vi "plate tap.vi"() -> ()   [LabVIEW 2014]
uses:
  <vilib>/userdefined/High Color/IMAQdx.ctl
  <vilib>/Utility/file.llb/Write To Spreadsheet File (DBL).vi
  <vilib>/Utility/file.llb/Write To Spreadsheet File (string).vi
  <vilib>/vision/driver/NI_Vision_Acquisition_Software.lvlib
panel:
  in  "Tags":string
  in  "Hold Time (frames)":i32
  in  "ISI  (frames)":i32
  in  "Array":dbl[](array[numeric])
  in  "Trials Per Voltage":i32
  in  "Start Recording":bool
  in  "Min Voltage":dbl
  out "Frames":i32
  out "Error":string
  out "Save Directory":path
  out "Buffer Number Out":u32
  out "Image":T1(plugin-control)
  in  "stop":bool
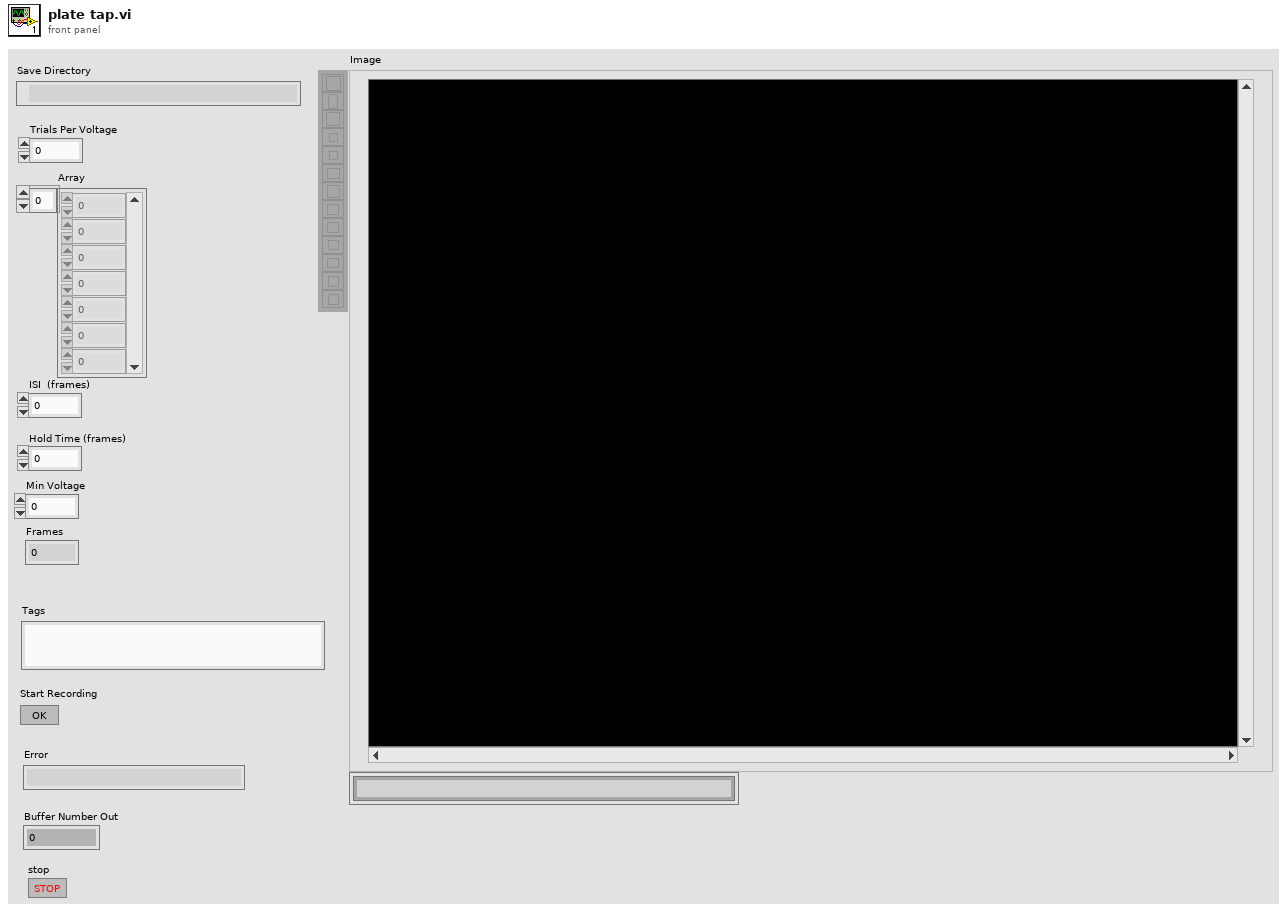
[diagram p1: front panel]
types:
  T1 = typedef "IMAQ Image.ctl" = refnum<image>
  T2 = typedef "IMAQdx.ctl" = refnum<k21>
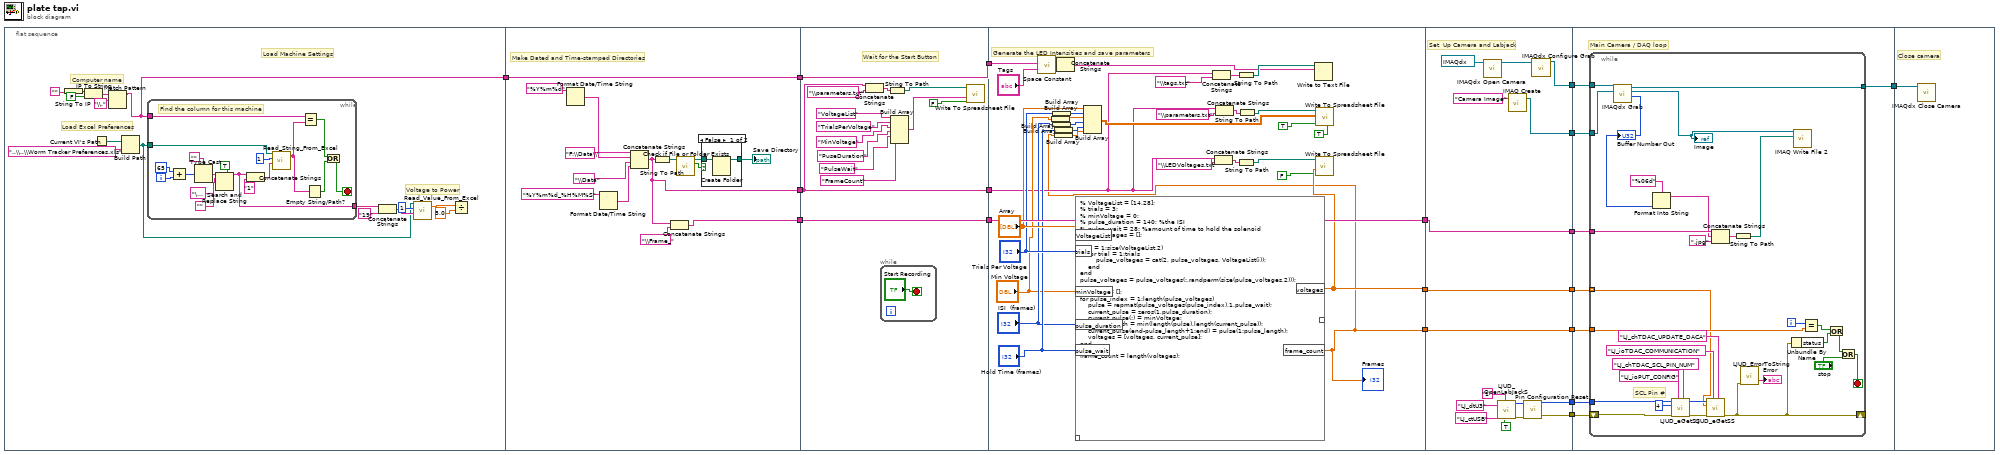
[diagram p0: block diagram]
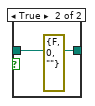
[diagram p2: hidden frame]
diagram:
  n1 = flat-sequence {
    tunnel: [w19] -> w2
    tunnel: [w55] -> w8
    tunnel: [w53] -> w6
    tunnel: [w52] -> w3
    tunnel: w2 -> [w52]
    tunnel: w8 -> [w82]
    tunnel: [w82] -> w7
    tunnel: w6 -> [w77]
    tunnel: [w77] -> w5
    tunnel: [w69] -> w4
    tunnel: w3 -> [w69]
    tunnel: w7 -> [w112]
    tunnel: [w112] -> w13
    tunnel: [w110] -> w11
    tunnel: [w84] -> w10
    tunnel: w5 -> [w86]
    tunnel: w4 -> [w85]
    tunnel: w13 -> [w125]
    tunnel: [w127] -> w18
    tunnel: [w126] -> w17
    tunnel: [w125] -> w16
    tunnel: [w115] -> w14
    tunnel: [w124] -> w12
    tunnel: w11 -> [w124]
    tunnel: w10 -> [w123]
    tunnel: [w123] -> w9
    tunnel: [w116] -> w1
    tunnel: w18 -> [w138]
    tunnel: w17 -> [w137]
    tunnel: w16 -> [w136]
    tunnel: [w135] -> w15
    tunnel: w14 -> [w134]
    tunnel: w12 -> [w132]
    tunnel: w9 -> [w131]
    tunnel: w1 -> [w133]
    tunnel: w15 -> [w169]
    frame #0 {
      # "Voltage to Power"
      # "Load Excel Preferences"
      # "Computer name"
      # "Load Machine Settings"
      n2 = String To IP(1:"") -> (0:w33:u32)
      n3 = IP To String(1:FALSE, 2:w33) -> (0:w30:string)
      n4 = Current VI's Path() -> (path=w28:path)
      n5 = Match Pattern(string=w30, regular expression="\\.") -> (before substring=w19:string)  [unwired: 1 in, 3 out]
      n6 = Build Path(base path=w28, name or relative path="..\\..\\Worm Tracker Preferences.xls") -> (appended path=w22:path)
      n7 = while {
        tunnel: w22 -> [w46]
        tunnel: w19 -> [w43]
        tunnel: [w34] -> w26
        i -> [w51]
        stop <- w40 stop-if-true
        # "Find the column for this machine"
        n8 = Add(x=65, y=w51) -> (x+y=w49:i32)
        n9 = Type Cast(type="", x=w49) -> (*(type *) &x=w35:string)
        n10 = Search and Replace String(replace all?=TRUE, input string=w35, search string="\u0000", replace string="") -> (result string=w34:string)  [unwired: 4 in, 3 out]
        n11 = Concatenate Strings(w34, "1") -> (w45:string)
        n12 = call "Read_String_From_Excel.vi"("Selected Cell"=w45, "Work Sheet"=1, "Excel File Path"=w46) -> ("Data from Cell"=w44:string)  [unwired: 1 in, 1 out]
        n13 = Equal?(x=w43, y=w44) -> (x = y?=w42:bool)
        n14 = Empty String/Path?(string/path=w44) -> (empty?=w41:bool)
        n15 = Or(x=w42, y=w41) -> (x .or. y?=w40:bool)
      }
      n16 = Concatenate Strings(w26, "19") -> (w24:string)
      n17 = call "Read_Value_From_Excel.vi"("Selected Cell"=w24, "Work Sheet"=1, "Excel File Path"=w22) -> ("Data from Cell"=w21:dbl)  [unwired: 1 in, 1 out]
      n18 = Divide(x=w21, y=5.0) -> ()  [unwired: 1 out]
    }
    frame #1 {
      # "Make Dated and Time-stamped Directories"
      n19 = Format Date/Time String(time format string (%c)="%Y%m%d") -> (date/time string=w56:string)  [unwired: 2 in]
      n20 = Format Date/Time String(time format string (%c)="%Y%m%d_%H%M%S") -> (date/time string=w60:string)  [unwired: 2 in]
      n21 = Concatenate Strings("F:\\Data\\", w56, "\\Data", w60) -> (w53:string)
      n22 = String To Path(string=w53) -> (path=w59:path)
      n23 = Concatenate Strings(w53, "\\Frame_") -> (w55:string)
      n24 = call <vilib>:"Check if File or Folder Exists.vi"("path"=w59) -> ("file or folder exists?"=w64:bool, "dup path"=w63:path)  [unwired: 8 in, 1 out]
      n25 = case shown="False" w64 {
        tunnel: [w66 w68] -> w58
        tunnel: w63 -> [w67 w68]
        frame False {
          n26 = Create Folder(path (use dialog)=w67) -> (created path=w66:path)  [unwired: 2 in, 2 out]
        }
        frame True {
          (unwired) errorcluster {"status"=FALSE, "code"=0, "source"=""} ("error out")
        }
      }
      "Save Directory" <- w58
    }
    frame #2 {
      # "Wait for the Start Button"
      n27 = Concatenate Strings(w77, "\\parameters.txt") -> (w81:string)
      n28 = while {
        stop <- "Start Recording" stop-if-true
      }
      n29 = String To Path(string=w81) -> (path=w80:path)
      n30 = Build Array("VoltageList", "TrialsPerVoltage", "MinVoltage", "PuseDuration", "PulseWait", "FrameCount") -> (w75:string[])
      n31 = call-poly <vilib>:"Write To Spreadsheet File.vi"("append to file? (new file:F)"=FALSE, "1D data"=w75, "file path (dialog if empty)"=w80) -> ()  [unwired: 5 in, 1 out]
    }
    frame #3 {
      # "Generate the LED Intensities and save parameters"
      n32 = call <vilib>:"Space Constant.vi"() -> ("String"=w88:string)
      n33 = Build Array("Min Voltage") -> (w93:dbl[])
      n34 = Build Array("Trials Per Voltage") -> (w102:i32[])
      n35 = Build Array("ISI  (frames)") -> (w95:i32[])
      n36 = Build Array("Hold Time (frames)") -> (w97:i32[])
      n37 = Concatenate Strings(w85, w88, "Tags") -> (w87:string)
      n38 = script code="% VoltageList = [14,28];\n% trials = 3;\n% minVoltage = 0;\n% pulse_duration = 140; %the ISI\n% pulse_wait = 28; %amount of time to hold the solenoid\npulse_voltages = [];\n\nfor i = 1:size(VoltageList,2)\n    for trial = 1:trials\n        pulse_voltages = cat(2, pulse_voltages, VoltageList(i));\n    end\nend\npulse_voltages = pulse_voltages(:,randperm(size(pulse_voltages,2)));\n\nvoltages = [];\nfor pulse_index = 1:length(pulse_voltages)\n    pulse = repmat(pulse_voltages(pulse_index),1,pulse_wait);\n    current_pulse = zeros(1,pulse_duration);\n    current_pulse(:) = minVoltage;\n    pulse_length = min(length(pulse),length(current_pulse));\n    current_pulse(end-pulse_length+1:end) = pulse(1:pulse_length);\n    voltages = [voltages, current_pulse];\nend\n\nframe_count = length(voltages);"("pulse_duration"="ISI  (frames)", "trials"="Trials Per Voltage", "minVoltage"="Min Voltage", "VoltageList"="Array", "pulse_wait"="Hold Time (frames)") -> ("voltages"=w110:dbl[], "frame_count"=w84:dbl)  [unwired: 1 in, 1 out]
      "Frames" <- w84
      n39 = Build Array(w84) -> (w99:dbl[])
      n40 = Build Array("Array", w102, w93, w95, w97, w99) -> (w100:dbl[][])
      n41 = Concatenate Strings(w86, "\\tags.txt") -> (w91:string)
      n42 = Concatenate Strings(w86, "\\LEDVoltages.txt") -> (w114:string)
      n43 = Concatenate Strings(w86, "\\parameters.txt") -> (w108:string)
      n44 = String To Path(string=w91) -> (path=w90:path)
      n45 = String To Path(string=w114) -> (path=w113:path)
      n46 = String To Path(string=w108) -> (path=w107:path)
      n47 = Write to Text File(file (use dialog)=w90, text=w87) -> ()  [unwired: 2 in, 3 out]
      n48 = call-poly <vilib>:"Write To Spreadsheet File.vi"("append to file? (new file:F)"=FALSE, "1D data"=w110, "file path (dialog if empty)"=w113) -> ()  [unwired: 5 in, 1 out]
      n49 = call-poly <vilib>:"Write To Spreadsheet File.vi"("transpose? (no:F)"=TRUE, "append to file? (new file:F)"=TRUE, "2D data"=w100, "file path (dialog if empty)"=w107) -> ()  [unwired: 4 in, 1 out]
    }
    frame #4 {
      # "Set  Up Camera and Labjack"
      n50 = call <vilib>:"IMAQdx Open Camera.vi"("Session In"=T2 "cam0") -> ("Session Out"=w129:T2)  [unwired: 9 in, 1 out]
      n51 = call "LJUD_OpenLabJackS.vi"("FirstFound"=TRUE, "Address"="1" ("DeviceType"), "ConnectionType"="LJ_ctUSB", "DeviceType"="LJ_dtU3") -> ("error out"=w117:errorcluster, "Handle"=w118:i32)  [unwired: 5 in, 1 out]
      n52 = call "IMAQ Create"("Image Name"="Camera Image") -> ("New Image"=w126:T1)  [unwired: 4 in, 1 out]
      n53 = call "Pin Configuration Reset.vi"("error in"=w117, "Handle In"=w118) -> ("error out"=w116:errorcluster, "Handle Out"=w115:i32)  [unwired: 8 in]
      n54 = call <vilib>:"IMAQdx Configure Grab.vi"("Session In"=w129) -> ("Session Out"=w127:T2)  [unwired: 9 in, 1 out]
    }
    frame #5 {
      # "Main Camera / DAQ loop"
      n55 = while {
        tunnel: w138 -> [w168]
        tunnel: [w167] -> w135
        tunnel: w137 -> [w166]
        tunnel: w136 -> [w164]
        tunnel: w134 -> [w140]
        shift-right: [w141] -> _
        shift-left: w133 -> [w142]
        tunnel: w132 -> [w139] mode=indexing
        tunnel: w131 -> [w150]
        i -> [w151]
        stop <- w157 stop-if-true
        # "SCL Pin #"
        n56 = call <vilib>:"IMAQdx Grab.vi"("Image In"=w166, "Session In"=w168) -> ("Buffer Number Out"=w160:u32, "Image Out"=w165:T1, "Session Out"=w167:T2)  [unwired: 6 in, 1 out]
        "Image" <- w165
        "Buffer Number Out" <- w160
        n57 = Format Into String(format string="%06d" ("string"), w160) -> (resulting string=w159:string)  [unwired: 2 in, 1 out]
        n58 = call "LJUD_eGetSS.vi"("Channel"="LJ_chTDAC_SCL_PIN_NUM", "IOType"="LJ_ioPUT_CONFIG", "error in"=w142, "Value Write"=4, "Handle In"=w140) -> ("error out"=w143:errorcluster, "Handle Out"=w146:i32)  [unwired: 4 in, 1 out]
        n59 = call "LJUD_eGetSS.vi"("Channel"="LJ_chTDAC_UPDATE_DACA", "IOType"="LJ_ioTDAC_COMMUNICATION", "error in"=w143, "Value Write"=w139, "Handle In"=w146) -> ("error out"=w141:errorcluster)  [unwired: 4 in, 2 out]
        n60 = Concatenate Strings(w164, w159, ".jpg" ("string")) -> (w162:string)
        n61 = String To Path(string=w162) -> (path=w161:path)
        n62 = call "LJUD_ErrorToString.vi"("error in"=w141) -> ("String"=→"Error":string)  [unwired: 10 in]
        n63 = Unbundle By Name(w141) -> ("status"=w154:bool)
        n64 = call-poly "IMAQ Write File 2"("File Path"=w161, "Image"=w165) -> ()  [unwired: 8 in, 2 out]
        n65 = Equal?(x=w151, y=w150) -> (x = y?=w153:bool)
        n66 = Or(x=w153, y=w154) -> (x .or. y?=w152:bool)
        n67 = Or(x=w152, y="stop") -> (x .or. y?=w157:bool)
      }
    }
    frame #6 {
      # "Close camera"
      n68 = call <vilib>:"IMAQdx Close Camera.vi"("Session In"=w169) -> ()  [unwired: 10 in, 1 out]
    }
  }
